vi "terminate.vi"(8 "error in (no error)":errorcluster, 11 "ScanModeTS090821Circular2D in":refnum<class "ImagingModeTS090821Circular2D.lvclass">) -> (0 "error out":errorcluster, 3 "ScanModeTS090821Circular2D out":refnum<class "ImagingModeTS090821Circular2D.lvclass">)   [LabVIEW 2010, in "ImagingModeTS090821Circular2D.lvclass"]
doc: "The dynamic dispatch version of this VI terminates the plug-in object by releasing all of its resources."
uses:
  ImagingModeTS090821Circular2D.lvclass
  ImagingModeTS090821Circular2D.lvclass/ImagingModeTS090821Circular2D.ctl
  common/classes/Image/Image/Image.lvclass
  ImagingModeDL091001Scaffold/ImagingModeDL091001Scaffold/ImagingModeDL091001Scaffold.lvclass
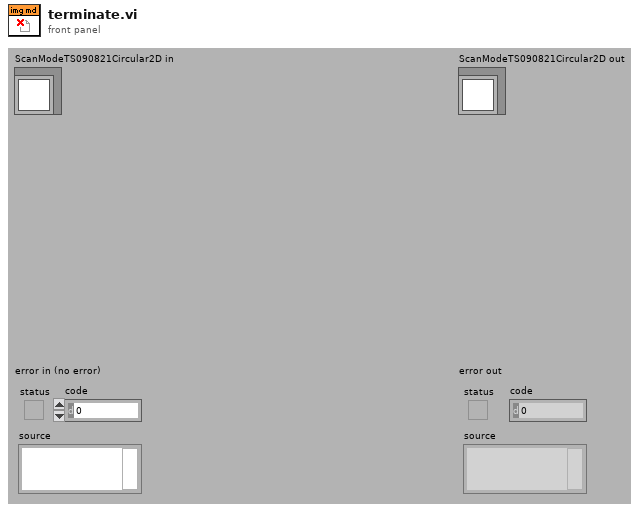
[diagram p1: front panel]
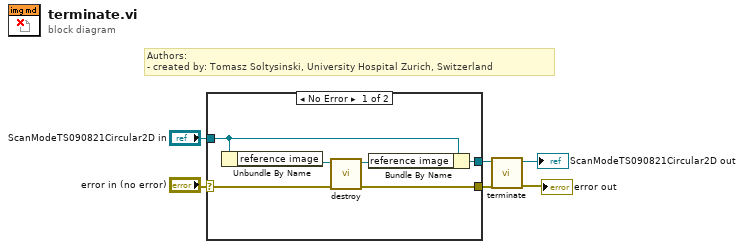
[diagram p0: block diagram]
diagram:
  # "Authors: \n- created by: Tomasz Soltysinski, University Hospital Zurich, Switzerland"
  n1 = case shown="No Error" "error in (no error)" {
    selector: "error in (no error)" -> [w12 w13]
    tunnel: [w11 w13] -> w5
    tunnel: "ScanModeTS090821Circular2D in" -> [w8 w14]
    tunnel: [w7 w14] -> w3
    frame No Error {
      n2 = Unbundle By Name(w8) -> ("reference image"=w10:refnum<class "Image.lvclass">)
      n3 = call-dynamic "destroy.vi"("error in (no error)"=w12, "Image in"=w10) -> ("error out"=w11:errorcluster, "Image out"=w9:refnum<class "Image.lvclass">)  [unwired: 8 in]
      n4 = Bundle By Name(cluster=w8, "reference image"=w9) -> (w7:refnum<class "ImagingModeTS090821Circular2D.lvclass">)
    }
    frame Error {
    }
  }
  n5 = call-parent "terminate.vi"("error in (no error)"=w5, "GenericPlugin in"=w3) -> ("error out"=→"error out":errorcluster, "GenericPlugin out"=→"ScanModeTS090821Circular2D out":refnum<class "ImagingModeTS090821Circular2D.lvclass">)  [unwired: 8 in]
